vi "PPCS_TRAJECTORY_CMD_FOLLOW_SWERVE.vi"(6 "Pass_Through_Time":dbl=-1.0 format="%33.4f", 8 "Init":bool) -> (0 "AtReference":bool, 1 "Complete":bool, 3 "Chassis Velocity Target SI":T1 {"vOmega" format="%10.3f"; "vY" format="%10.3f"; "vX" format="%10.3f"})   [LabVIEW 2019]
uses:
  <vilib>/Rock Robotics/WPI/ThirdParty/JAS_Junk/TrajLib/Trajectory_Library.lvlib
  PPCS_TRAJECTORY_GLOBALS.vi
  <vilib>/Rock Robotics/WPI/ThirdParty/MJansen/PathPlanner/PathPlanner24.lvlib
  <vilib>/Rock Robotics/WPI/ThirdParty/JAS_Junk/TrajLib/TypeDef/CHASSIS_SPEEDS.ctl
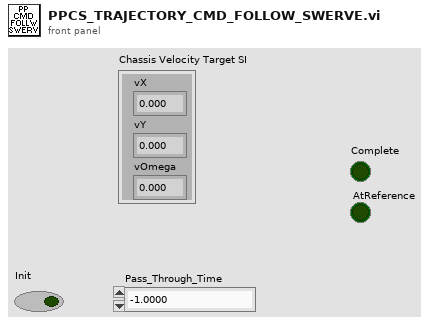
[diagram p1: front panel]
types:
  T1 = typedef "Trajectory_Library.lvlib/CHASSIS_SPEEDS.ctl" = cluster{"vX":dbl, "vY":dbl, "vOmega":dbl}
  T2 = typedef "PathPlanner24.lvlib/PathPlannerPath.ctl" = cluster{"Reversed":bool, "RotationTargets":T3[], "ConstraintZones":T5[], "EventMarkers":T7[], "GlobalConstraints":T6, "GoalEndState":T10, "AllPoints":T11[], "Name":string, "Waypoints":T13[], "PointTowardsZones":T14[], "IdealStartingState":T15, "IsChoreoPath":bool, "PreventFlipping":bool}
  T3 = typedef "PathPlanner24.lvlib/PathPlannerRotationTarget.ctl" = cluster{"position":dbl, "rotation":T4, "Exists":bool}
  T4 = typedef "Trajectory_Library.lvlib/ROTATION2D.ctl" = cluster{"VALUE":dbl, "COS":dbl, "SIN":dbl}
  T5 = typedef "PathPlanner24.lvlib/PathPlannerConstraintsZone.ctl" = cluster{"minPosition":dbl, "maxPosition":dbl, "Constraints":T6, "Present":bool}
  T6 = typedef "PathPlanner24.lvlib/PathPlannerPathConstraints.ctl" = cluster{"MaxVelocityMps;":dbl, "MaxAccelerationMpsSq;":dbl, "MaxAngularVelRadPsEc;":dbl, "MaxAngularAccRadPSecSq":dbl, "Exists":bool, "Unlimited":bool, "NominalVoltageVolts":dbl}
  T7 = typedef "PathPlanner24.lvlib/PathPlannerEventMarker.ctl" = cluster{"Position":dbl, "Command":T8, "TriggerName":string, "EndPosition":dbl}
  T8 = typedef "PathPlanner24.lvlib/PathPlannerCommandUtil.ctl" = cluster{"waitTime":dbl, "name":string, "pathName":string, "commands":cluster{"type":T9, "waitTime":dbl, "name":string, "pathName":string}[], "type":T9}
  T9 = typedef "PathPlanner24.lvlib/PathPlanner_CommandUtilType_ENUM.ctl" = enum16{"Unknown", "Wait", "Named", "Path", "Sequential", "Parallel", "Race", "Deadline"}
  T10 = typedef "PathPlanner24.lvlib/PathPlannerGoalEndState.ctl" = cluster{"VelocityMPS":dbl, "Rotation":T4}
  T11 = typedef "PathPlanner24.lvlib/PathPlannerPathPoint.ctl" = cluster{"Position":T12, "DistAlongPath":dbl, "MaxV":dbl, "Constraints":T6, "RotationTarget":T3, "WaypointRelativePos":dbl}
  T12 = typedef "Trajectory_Library.lvlib/TRANSLATION2D.ctl" = cluster{"X":dbl, "Y":dbl}
  T13 = typedef "PathPlanner24.lvlib/PathPlannerWaypoint.ctl" = cluster{"prevControl":T12, "anchor":T12, "nextControl":T12, "PrevExists":bool, "NextExists":bool}
  T14 = typedef "PathPlanner24.lvlib/PathPlannerPointTowardsZone.ctl" = cluster{"RotationOffset":T4, "Name":string, "TargetPosition":T12, "MinPosition":dbl, "MaxPosition":dbl}
  T15 = typedef "PathPlanner24.lvlib/PathPlannerIdealStartingState.ctl" = cluster{"VelocityMPS":dbl, "Rotation":T4}
  T16 = typedef "Trajectory_Library.lvlib/PID_TUNING.ctl" = cluster{"Kp":dbl, "Ki":dbl, "Kd":dbl, "MaximumIntegral":dbl, "MinimumIntegral":dbl, "IntegralZone":dbl}
  T17 = typedef "Trajectory_Library.lvlib/POSE2D.ctl" = cluster{"TRANSLATION":T12, "ROTATION":T4}
  T18 = typedef "Trajectory_Library.lvlib/PROFILED_PID_CONTROLLER.ctl" = cluster{"Controller":T19, "Goal":T20, "Setpoint":T20, "Constraint":T21}
  T19 = typedef "Trajectory_Library.lvlib/PID_CONTROLLER.ctl" = cluster{"Kp":dbl, "Ki":dbl, "Kd":dbl, "Period":dbl, "Max_Integral":dbl, "Min_Integral":dbl, "Max_Input":dbl, "Min_Input":dbl, "Continuous":bool, "PositionError":dbl, "VelocityError":dbl, "PrevError":dbl, "Total_Integral":dbl, "PositionTolerance":dbl, "VelocityTolerance":dbl, "SetPoint":dbl, "Kf":dbl, "Prev_Deriv":dbl, "Prev_Deriv 2":dbl, "DerivativeFilter":bool, "Min_Output":dbl, "Max_Output":dbl, "Prev_F_P":dbl, "Prev_F_P_2":dbl, "AntiWindupActive":bool, "Measurement":dbl, "IntegralZone":dbl}
  T20 = typedef "Trajectory_Library.lvlib/TRAPEZOID_PROFILE_STATE.ctl" = cluster{"Position":dbl, "Velocity":dbl}
  T21 = typedef "Trajectory_Library.lvlib/TRAPEZOID_PROFILE_CONSTRAINT.ctl" = cluster{"MaxVelocity":dbl, "MaxAcceleration":dbl}
  T22 = typedef "Trajectory_Library.lvlib/HOLONOMIC_PACK_TUNING.ctl" = cluster{"X PID Tuning":T16, "Y PID Tuning":T16, "thetaProfiledPID_CTRL":T18}
  T23 = typedef "PathPlanner24.lvlib/PathPlannerCmdFollowHolConfig.ctl" = cluster{"HOLONOMIC_CTRL_PACK_TUNING":T22, "Max Wheel Speed M/S":dbl, "Tolerance SI":T17, "Drive Base Radius M":dbl, "ControlPastEnd_Sec":dbl, "Period_Sec":dbl, "Trigger Events":bool}
  T24 = typedef "Trajectory_Library.lvlib/HOLONOMIC_DRV_CTRL.ctl" = cluster{"poseTolerance":T17, "poseError":T17, "Enabled":bool, "PID_xCtrl":T19, "PID_yCtrl":T19, "PROF_PID_thetaCtrl":T18, "RotationError":T4, "FirstRun":bool}
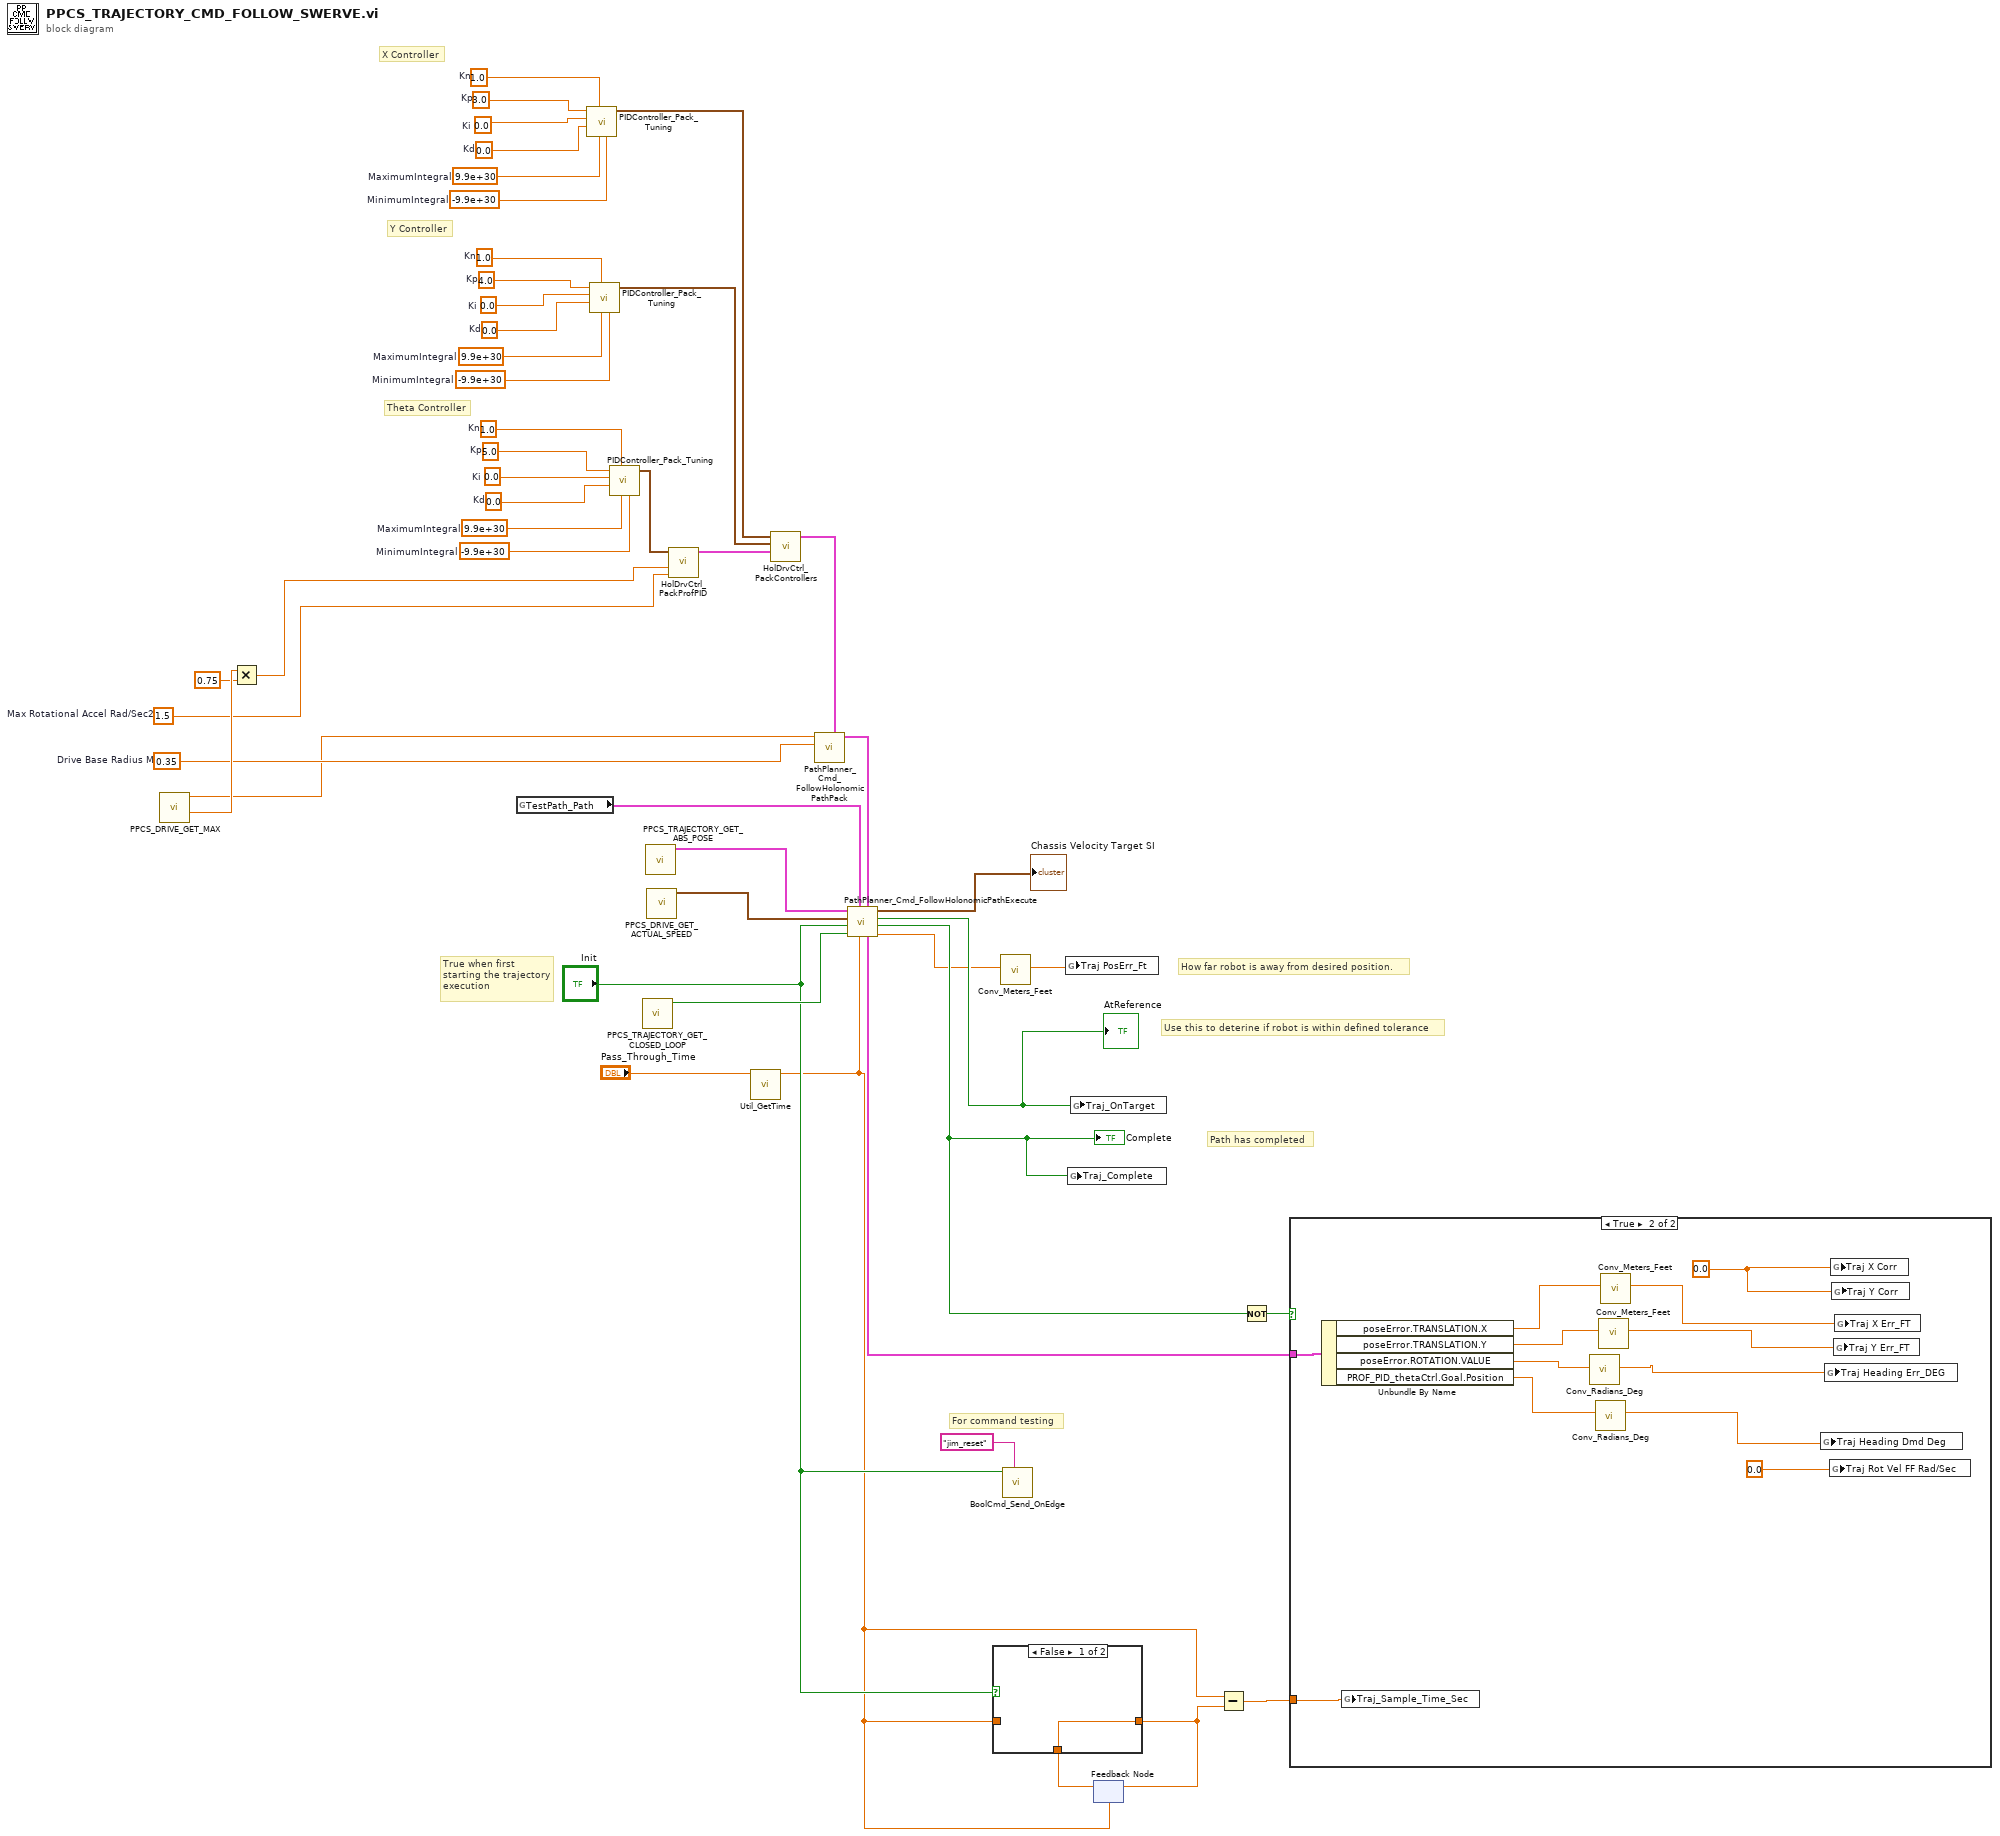
[diagram p0: block diagram]
diagram:
  w38 = 1.0  # Kn
  w35 = 5.0  # Kp
  w26 = 0.0  # Ki
  w25 = 0.0  # Kd
  w24 = 9.9e+30  # MaximumIntegral
  w23 = -9.9e+30  # MinimumIntegral
  w40 = 1.0  # Kn
  w37 = 3.0  # Kp
  w34 = 0.0  # Ki
  w33 = 0.0  # Kd
  w32 = 9.9e+30  # MaximumIntegral
  w31 = -9.9e+30  # MinimumIntegral
  w39 = 1.0  # Kn
  w36 = 4.0  # Kp
  w30 = 0.0  # Ki
  w29 = 0.0  # Kd
  w28 = 9.9e+30  # MaximumIntegral
  w27 = -9.9e+30  # MinimumIntegral
  w20 = 0.35  # Drive Base Radius M
  w21 = 1.5  # Max Rotational Accel Rad/Sec2
  # "For command testing"
  # "Path has completed"
  # "How far robot is away from desired position."
  # "Use this to deterine if robot is within defined tolerance"
  # "Theta Controller"
  # "Y Controller"
  # "X Controller"
  # "True when first\nstarting the trajectory\nexecution"
  n1 = call "PPCS_DRIVE_GET_MAX.vi"() -> ("Max Rotational Vel (Rad/Sec)"=w48:dbl, "Max Wheel Vel (Meter/Sec)"=w14:dbl)  [unwired: 10 in]
  n2 = Multiply(x=w48, y=0.75) -> (x*y=w22:dbl)
  n3 = global read "PPCS_TRAJECTORY_GLOBALS.vi" "TestPath_Path"() -> (w19:T2)
  n4 = call <vilib>:"PIDController_Pack_Tuning.vi"("MinimumIntegral"=w31, "MaximumIntegral"=w32, "Kn"=w40, "Kd"=w33, "Ki"=w34, "Kp"=w37) -> ("PID Tuning"=w44:T16)  [unwired: 5 in]
  n5 = call <vilib>:"PIDController_Pack_Tuning.vi"("MinimumIntegral"=w27, "MaximumIntegral"=w28, "Kn"=w39, "Kd"=w29, "Ki"=w30, "Kp"=w36) -> ("PID Tuning"=w45:T16)  [unwired: 5 in]
  n6 = call <vilib>:"PIDController_Pack_Tuning.vi"("MinimumIntegral"=w23, "MaximumIntegral"=w24, "Kn"=w38, "Kd"=w25, "Ki"=w26, "Kp"=w35) -> ("PID Tuning"=w41:T16)  [unwired: 5 in]
  n7 = call "PPCS_TRAJECTORY_GET_CLOSED_LOOP.vi"() -> ("AUTO_CLOSED_LOOP"=w16:bool)  [unwired: 11 in]
  n8 = call "PPCS_TRAJECTORY_GET_ABS_POSE.vi"() -> ("Absolute Odometry Pose"=w18:T17)  [unwired: 11 in]
  n9 = call "PPCS_DRIVE_GET_ACTUAL_SPEED.vi"() -> ("Drv Chassis Actual Velocity"=w17:T1)  [unwired: 11 in]
  n10 = call <vilib>:"HolDrvCtrl_PackProfPID.vi"("Max Accel"=w21, "Max Speed"=w22, "Theta PID Tuning"=w41) -> ("Theta PID CONTROLLER"=w46:T18)  [unwired: 8 in]
  n11 = call <vilib>:"Util_GetTime.vi"("Pass_Through_Time"="Pass_Through_Time") -> ("FPGA_Time_Seconds"=w4:dbl)  [unwired: 8 in, 2 out]
  n12 = call <vilib>:"HolDrvCtrl_PackControllers.vi"("thetaProfiledPID_CTRL"=w46, "Y PID Tuning"=w45, "X PID Tuning"=w44) -> ("HOLONOMIC_CTRL_PACK_TUNING"=w43:T22)  [unwired: 8 in]
  n13 = call <vilib>:"PathPlanner_Cmd_FollowHolonomicPathPack.vi"("HOLONOMIC_CTRL_PACK_TUNING"=w43, "Drive Base Radius M"=w20, "Max Wheel Speed M/S"=w14) -> ("PathPlanner_Ctrl_HolDrvConfig"=w42:T23)  [unwired: 8 in]
  n14 = call <vilib>:"PathPlanner_Cmd_FollowHolonomicPathExecute.vi"("PathPlanner_Cmd_FollowHolConfig"=w42, "PassthroughTime_SEC"=w4, "PathPlannerPath"=w19, "Enabled"=w16, "Reset"="Init", "CurrentChassisSpeeds"=w17, "Current Pose SI"=w18) -> ("Position Error M"=w7:dbl, "Complete"=w9:bool, "At Reference"=w11:bool, "calcChassisSpeed"=→"Chassis Velocity Target SI":T1, "outHOLONOMIC_DRV_CTRL"=w12:T24)
  "AtReference" <- w11
  "Complete" <- w9
  n15 = call <vilib>:"Conv_Meters_Feet.vi"("Meters"=w7) -> ("Feet"=w8:dbl)  [unwired: 10 in]
  n16 = call <vilib>:"BoolCmd_Send_OnEdge.vi"("Command Name"="jim_reset", "Value"="Init") -> ()  [unwired: 9 in, 1 out]
  n17 = global write "PPCS_TRAJECTORY_GLOBALS.vi" "Traj PosErr_Ft"(w8) -> ()
  n18 = global write "PPCS_TRAJECTORY_GLOBALS.vi" "Traj_Complete"(w9) -> ()
  n19 = global write "PPCS_TRAJECTORY_GLOBALS.vi" "Traj_OnTarget"(w11) -> ()
  n20 = feedback #1(w4) -> (w2:dbl)
  n21 = case shown="False" "Init" {
    tunnel: w4 -> [_ w50]
    tunnel: [w49 w50] -> w3
    tunnel: w2 -> [w49 _]
    frame False {
    }
    frame True {
    }
  }
  n22 = feedback-in #1(w3) -> ()
  n23 = Subtract(x=w4, y=w3) -> (x-y=w1:dbl)
  n24 = Not(x=w9) -> (.not. x?=w10:bool)
  n25 = case shown="True" w10 {
    tunnel: w12 -> [_ w58]
    tunnel: w1 -> [_ w51]
    frame False {
    }
    frame True {
      w62 = 0.0 ("Y Corr")
      n26 = Unbundle By Name(w58) -> ("poseError.TRANSLATION.X"=w57:dbl, "poseError.TRANSLATION.Y"=w56:dbl, "poseError.ROTATION.VALUE"=w55:dbl, "PROF_PID_thetaCtrl.Goal.Position"=w53:dbl)
      n27 = global write "PPCS_TRAJECTORY_GLOBALS.vi" "Traj_Sample_Time_Sec"(w51) -> ()
      n28 = call <vilib>:"Conv_Radians_Deg.vi"("Radians"=w55) -> ("Degrees"=w54:dbl)  [unwired: 10 in]
      n29 = call <vilib>:"Conv_Radians_Deg.vi"("Radians"=w53) -> ("Degrees"=w52:dbl)  [unwired: 10 in]
      n30 = call <vilib>:"Conv_Meters_Feet.vi"("Meters"=w56) -> ("Feet"=w61:dbl)  [unwired: 10 in]
      n31 = call <vilib>:"Conv_Meters_Feet.vi"("Meters"=w57) -> ("Feet"=w60:dbl)  [unwired: 10 in]
      n32 = global write "PPCS_TRAJECTORY_GLOBALS.vi" "Traj Heading Dmd Deg"(w52) -> ()
      n33 = global write "PPCS_TRAJECTORY_GLOBALS.vi" "Traj Heading Err_DEG"(w54) -> ()
      n34 = global write "PPCS_TRAJECTORY_GLOBALS.vi" "Traj Rot Vel FF Rad/Sec"(0.0 ("Traj Heading Dmd Deg")) -> ()
      n35 = global write "PPCS_TRAJECTORY_GLOBALS.vi" "Traj X Corr"(w62) -> ()
      n36 = global write "PPCS_TRAJECTORY_GLOBALS.vi" "Traj Y Corr"(w62) -> ()
      n37 = global write "PPCS_TRAJECTORY_GLOBALS.vi" "Traj Y Err_FT"(w61) -> ()
      n38 = global write "PPCS_TRAJECTORY_GLOBALS.vi" "Traj X Err_FT"(w60) -> ()
    }
  }
